vi "fan_simulate.vi"() -> ()   [LabVIEW 2019]
panel:
  out "Ring":u16(ring)
  in  "LOWERING SPEED":dbl(knob) scale=0.0..10.0
  in  "?":bool
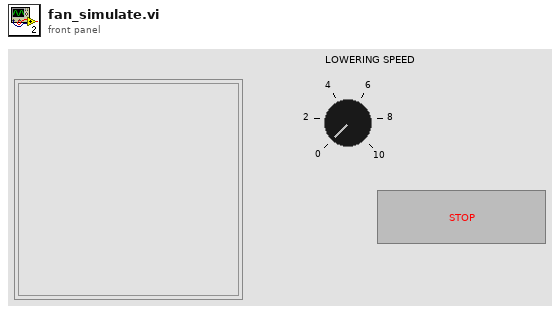
[diagram p1: front panel]
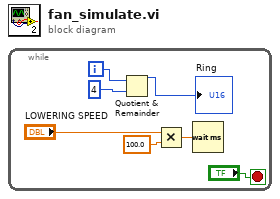
[diagram p0: block diagram]
diagram:
  n1 = while {
    i -> [w7]
    stop <- "?" stop-if-true
    n2 = Quotient & Remainder(x=w7, y=4) -> (x-y*floor(x/y)=→"Ring":i32)  [unwired: 1 out]
    n3 = Multiply(x="LOWERING SPEED", y=100.0) -> (x*y=w4:dbl)
    n4 = Wait (ms)(milliseconds to wait=w4) -> ()  [unwired: 1 out]
  }
